vi "Serial Convert.vi"(8 "Range (V)":sgl=20.0 format="%#_13g", 11 "Raw serial buffer":string="\u0000\u0000\u0000\u0000\u0000\u0000\u0000\u0000\u0000\u0000\u0000\u0000\u0000\u0000\u0000\u0000\u0000\u0000") -> (0 "V6 (V)":sgl, 1 "V5 (V)":sgl, 2 "V4 (V)":sgl, 3 "V3 (V)":sgl, 4 "V7 (V)":sgl, 5 "V2 (V)":sgl, 6 "V8 (V)":sgl, 7 "V1 (V)":sgl)   [LabVIEW 2014]
panel:
  # "PN 20/11/2014"
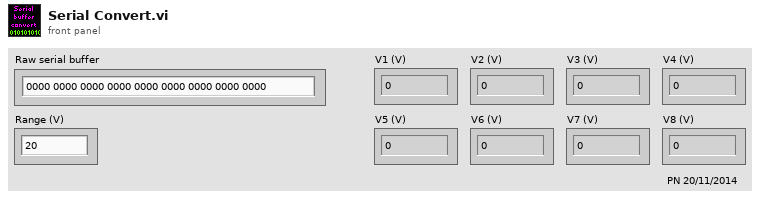
[diagram p1: front panel]
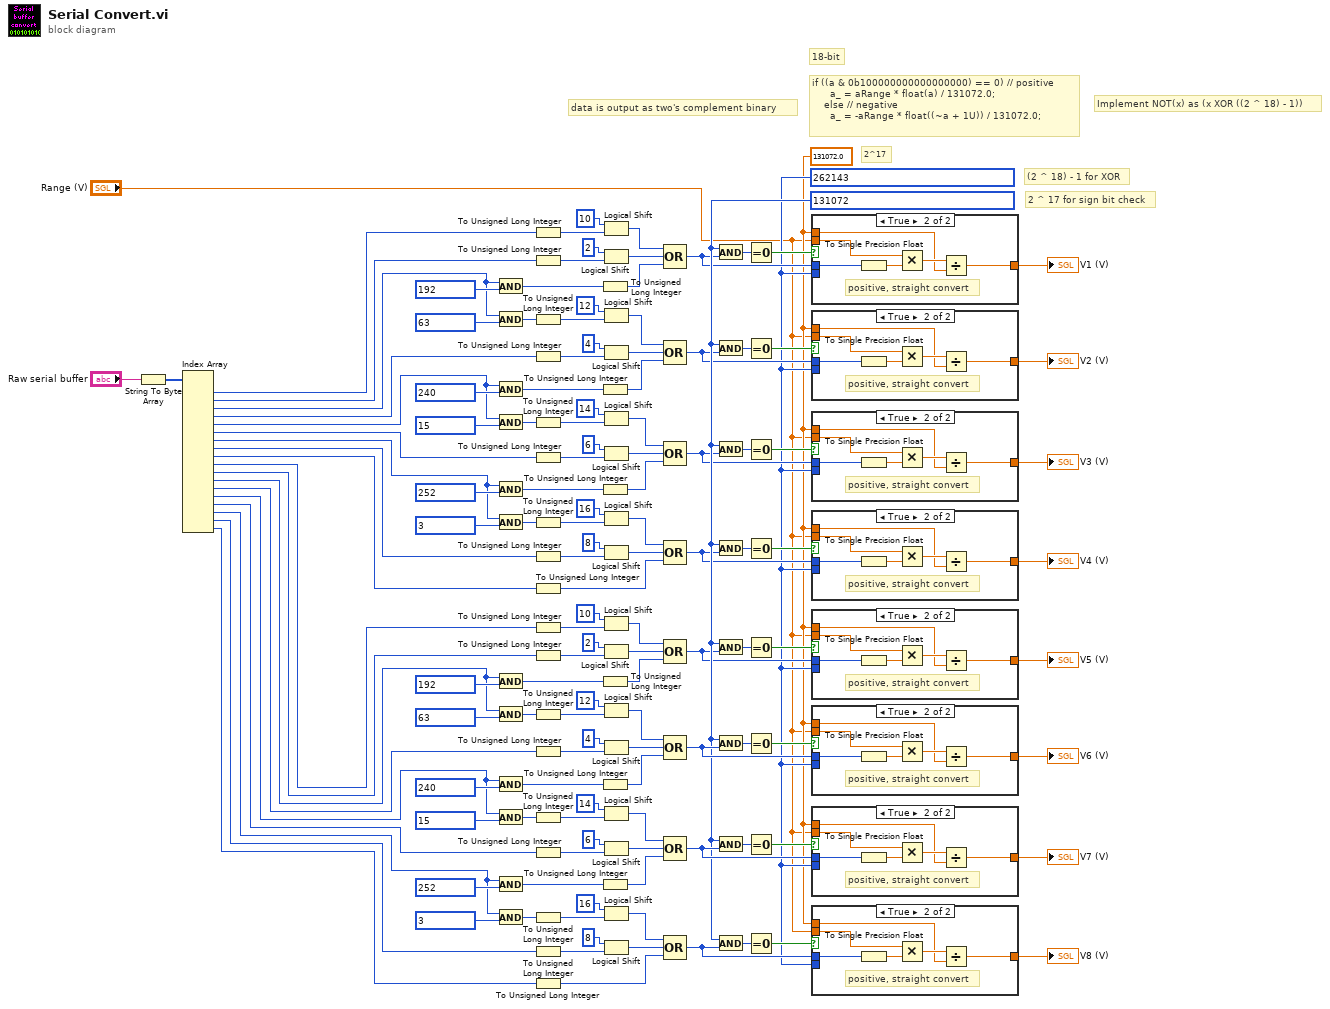
[diagram p0: block diagram]
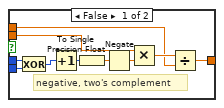
[diagram p2: hidden frame]
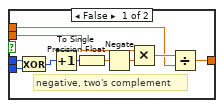
[diagram p3: hidden frame]
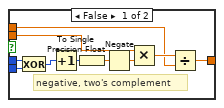
[diagram p4: hidden frame]
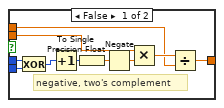
[diagram p5: hidden frame]
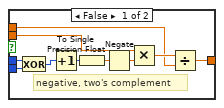
[diagram p6: hidden frame]
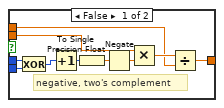
[diagram p7: hidden frame]
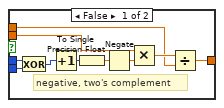
[diagram p8: hidden frame]
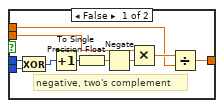
[diagram p9: hidden frame]
diagram:
  w3 = u32 262143
  w2 = sgl 131072.0
  w31 = u32 131072
  # "2 ^ 17 for sign bit check"
  # "(2 ^ 18) - 1 for XOR"
  # "Implement NOT(x) as (x XOR ((2 ^ 18) - 1))"
  # "18-bit"
  # "2^17"
  # "data is output as two's complement binary"
  # "if ((a & 0b100000000000000000) == 0) // positive\n      a_ = aRange * float(a) / 131072.0; \n    else // negative\n      a_ = -aRange * float((~a + 1U)) / 131072.0;"
  n1 = String To Byte Array(string="Raw serial buffer") -> (unsigned byte array=w131:u8[])
  n2 = Index Array(array=w131) -> (element #1=w135:u8, element #2=w132:u8, element #3=w122:u8, element #4=w118:u8, element #5=w109:u8, element #6=w104:u8, element #7=w96:u8, element #8=w91:u8, element #9=w87:u8, element #10=w30:u8, element #11=w29:u8, element #12=w28:u8, element #13=w27:u8, element #14=w26:u8, element #15=w25:u8, element #16=w24:u8, element #17=w23:u8, element #18=w22:u8)  [unwired: 18 in]
  n3 = And(x=w122, y=u8 192) -> (x .and. y?=w127:u8)
  n4 = And(x=w122, y=u8 63) -> (x .and. y?=w121:u8)
  n5 = And(x=w109, y=u8 240) -> (x .and. y?=w114:u8)
  n6 = And(x=w109, y=u8 15) -> (x .and. y?=w108:u8)
  n7 = And(x=w96, y=u8 252) -> (x .and. y?=w99:u8)
  n8 = And(x=w96, y=u8 3) -> (x .and. y?=w95:u8)
  n9 = And(x=w28, y=u8 192) -> (x .and. y?=w37:u8)
  n10 = And(x=w28, y=u8 63) -> (x .and. y?=w42:u8)
  n11 = And(x=w26, y=u8 240) -> (x .and. y?=w48:u8)
  n12 = And(x=w26, y=u8 15) -> (x .and. y?=w53:u8)
  n13 = And(x=w24, y=u8 252) -> (x .and. y?=w61:u8)
  n14 = And(x=w24, y=u8 3) -> (x .and. y?=w64:u8)
  n15 = To Unsigned Long Integer(number=w135) -> (unsigned 32bit integer=w130:u32)
  n16 = To Unsigned Long Integer(number=w132) -> (unsigned 32bit integer=w129:u32)
  n17 = To Unsigned Long Integer(number=w121) -> (unsigned 32bit integer=w120:u32)
  n18 = To Unsigned Long Integer(number=w118) -> (unsigned 32bit integer=w117:u32)
  n19 = To Unsigned Long Integer(number=w108) -> (unsigned 32bit integer=w106:u32)
  n20 = To Unsigned Long Integer(number=w104) -> (unsigned 32bit integer=w102:u32)
  n21 = To Unsigned Long Integer(number=w95) -> (unsigned 32bit integer=w93:u32)
  n22 = To Unsigned Long Integer(number=w91) -> (unsigned 32bit integer=w89:u32)
  n23 = To Unsigned Long Integer(number=w87) -> (unsigned 32bit integer=w86:u32)
  n24 = To Unsigned Long Integer(number=w30) -> (unsigned 32bit integer=w34:u32)
  n25 = To Unsigned Long Integer(number=w29) -> (unsigned 32bit integer=w35:u32)
  n26 = To Unsigned Long Integer(number=w42) -> (unsigned 32bit integer=w43:u32)
  n27 = To Unsigned Long Integer(number=w27) -> (unsigned 32bit integer=w45:u32)
  n28 = To Unsigned Long Integer(number=w53) -> (unsigned 32bit integer=w55:u32)
  n29 = To Unsigned Long Integer(number=w25) -> (unsigned 32bit integer=w58:u32)
  n30 = To Unsigned Long Integer(number=w64) -> (unsigned 32bit integer=w66:u32)
  n31 = To Unsigned Long Integer(number=w23) -> (unsigned 32bit integer=w69:u32)
  n32 = To Unsigned Long Integer(number=w22) -> (unsigned 32bit integer=w71:u32)
  n33 = To Unsigned Long Integer(number=w127) -> (unsigned 32bit integer=w126:u32)
  n34 = To Unsigned Long Integer(number=w114) -> (unsigned 32bit integer=w111:u32)
  n35 = To Unsigned Long Integer(number=w99) -> (unsigned 32bit integer=w98:u32)
  n36 = To Unsigned Long Integer(number=w37) -> (unsigned 32bit integer=w38:u32)
  n37 = To Unsigned Long Integer(number=w48) -> (unsigned 32bit integer=w51:u32)
  n38 = To Unsigned Long Integer(number=w61) -> (unsigned 32bit integer=w62:u32)
  n39 = Logical Shift(y=i16 10, x=w130) -> (x << y=w124:u32)
  n40 = Logical Shift(y=i16 2, x=w129) -> (x << y=w125:u32)
  n41 = Logical Shift(y=i16 12, x=w120) -> (x << y=w113:u32)
  n42 = Logical Shift(y=i16 4, x=w117) -> (x << y=w112:u32)
  n43 = Logical Shift(y=i16 14, x=w106) -> (x << y=w105:u32)
  n44 = Logical Shift(y=i16 6, x=w102) -> (x << y=w101:u32)
  n45 = Logical Shift(y=i16 16, x=w93) -> (x << y=w92:u32)
  n46 = Logical Shift(y=i16 8, x=w89) -> (x << y=w88:u32)
  n47 = Logical Shift(y=i16 10, x=w34) -> (x << y=w40:u32)
  n48 = Logical Shift(y=i16 2, x=w35) -> (x << y=w39:u32)
  n49 = Logical Shift(y=i16 12, x=w43) -> (x << y=w49:u32)
  n50 = Logical Shift(y=i16 4, x=w45) -> (x << y=w50:u32)
  n51 = Logical Shift(y=i16 14, x=w55) -> (x << y=w56:u32)
  n52 = Logical Shift(y=i16 6, x=w58) -> (x << y=w59:u32)
  n53 = Logical Shift(y=i16 16, x=w66) -> (x << y=w67:u32)
  n54 = Logical Shift(y=i16 8, x=w69) -> (x << y=w70:u32)
  n55 = Compound Arithmetic op=OR(w124, w125, w126) -> (w16:u32)
  n56 = Compound Arithmetic op=OR(w113, w112, w111) -> (w5:u32)
  n57 = Compound Arithmetic op=OR(w105, w101, w98) -> (w8:u32)
  n58 = Compound Arithmetic op=OR(w92, w88, w86) -> (w7:u32)
  n59 = Compound Arithmetic op=OR(w40, w39, w38) -> (w4:u32)
  n60 = Compound Arithmetic op=OR(w49, w50, w51) -> (w80:u32)
  n61 = Compound Arithmetic op=OR(w56, w59, w62) -> (w81:u32)
  n62 = Compound Arithmetic op=OR(w67, w70, w71) -> (w21:u32)
  n63 = And(x=w31, y=w16) -> (x .and. y?=w85:u32)
  n64 = And(x=w31, y=w5) -> (x .and. y?=w84:u32)
  n65 = And(x=w31, y=w8) -> (x .and. y?=w83:u32)
  n66 = And(x=w31, y=w7) -> (x .and. y?=w82:u32)
  n67 = And(x=w31, y=w4) -> (x .and. y?=w72:u32)
  n68 = And(x=w31, y=w80) -> (x .and. y?=w73:u32)
  n69 = And(x=w31, y=w81) -> (x .and. y?=w74:u32)
  n70 = And(x=w31, y=w21) -> (x .and. y?=w79:u32)
  n71 = Equal To 0?(x=w85) -> (x = 0?=w17:bool)
  n72 = Equal To 0?(x=w84) -> (x = 0?=w6:bool)
  n73 = Equal To 0?(x=w83) -> (x = 0?=w15:bool)
  n74 = Equal To 0?(x=w82) -> (x = 0?=w10:bool)
  n75 = Equal To 0?(x=w72) -> (x = 0?=w9:bool)
  n76 = Equal To 0?(x=w73) -> (x = 0?=w75:bool)
  n77 = Equal To 0?(x=w74) -> (x = 0?=w76:bool)
  n78 = Equal To 0?(x=w79) -> (x = 0?=w20:bool)
  n79 = case shown="True" w17 {
    tunnel: "Range (V)" -> [w143 w150]
    tunnel: w2 -> [w142 w148]
    tunnel: w16 -> [w138 w152]
    tunnel: [w141 w147] -> w18
    tunnel: w3 -> [w137 _]
    frame False {
      # "negative, two's complement"
      n80 = Exclusive Or(1:w137, 2:w138) -> (0:w139:u32)
      n81 = Increment(x=w139) -> (x+1=w144:u32)
      n82 = To Single Precision Float(number=w144) -> (single precision float=w146:sgl)
      n83 = Negate(x=w146) -> (-x=w140:sgl)
      n84 = Multiply(x=w143, y=w140) -> (x*y=w145:sgl)
      n85 = Divide(x=w145, y=w142) -> (x/y=w141:sgl)
    }
    frame True {
      # "positive, straight convert"
      n86 = To Single Precision Float(number=w152) -> (single precision float=w151:sgl)
      n87 = Multiply(x=w150, y=w151) -> (x*y=w149:sgl)
      n88 = Divide(x=w149, y=w148) -> (x/y=w147:sgl)
    }
  }
  "V1 (V)" <- w18
  n89 = case shown="True" w6 {
    tunnel: "Range (V)" -> [w159 w166]
    tunnel: w2 -> [w158 w164]
    tunnel: w5 -> [w154 w168]
    tunnel: [w157 w163] -> w13
    tunnel: w3 -> [w153 _]
    frame False {
      # "negative, two's complement"
      n90 = Exclusive Or(1:w153, 2:w154) -> (0:w155:u32)
      n91 = Increment(x=w155) -> (x+1=w160:u32)
      n92 = To Single Precision Float(number=w160) -> (single precision float=w162:sgl)
      n93 = Negate(x=w162) -> (-x=w156:sgl)
      n94 = Multiply(x=w159, y=w156) -> (x*y=w161:sgl)
      n95 = Divide(x=w161, y=w158) -> (x/y=w157:sgl)
    }
    frame True {
      # "positive, straight convert"
      n96 = To Single Precision Float(number=w168) -> (single precision float=w167:sgl)
      n97 = Multiply(x=w166, y=w167) -> (x*y=w165:sgl)
      n98 = Divide(x=w165, y=w164) -> (x/y=w163:sgl)
    }
  }
  "V2 (V)" <- w13
  n99 = case shown="True" w15 {
    tunnel: "Range (V)" -> [w175 w182]
    tunnel: w2 -> [w174 w180]
    tunnel: w8 -> [w170 w184]
    tunnel: [w173 w179] -> w14
    tunnel: w3 -> [w169 _]
    frame False {
      # "negative, two's complement"
      n100 = Exclusive Or(1:w169, 2:w170) -> (0:w171:u32)
      n101 = Increment(x=w171) -> (x+1=w176:u32)
      n102 = To Single Precision Float(number=w176) -> (single precision float=w178:sgl)
      n103 = Negate(x=w178) -> (-x=w172:sgl)
      n104 = Multiply(x=w175, y=w172) -> (x*y=w177:sgl)
      n105 = Divide(x=w177, y=w174) -> (x/y=w173:sgl)
    }
    frame True {
      # "positive, straight convert"
      n106 = To Single Precision Float(number=w184) -> (single precision float=w183:sgl)
      n107 = Multiply(x=w182, y=w183) -> (x*y=w181:sgl)
      n108 = Divide(x=w181, y=w180) -> (x/y=w179:sgl)
    }
  }
  "V3 (V)" <- w14
  n109 = case shown="True" w10 {
    tunnel: "Range (V)" -> [w191 w198]
    tunnel: w2 -> [w190 w196]
    tunnel: w7 -> [w186 w200]
    tunnel: [w189 w195] -> w12
    tunnel: w3 -> [w185 _]
    frame False {
      # "negative, two's complement"
      n110 = Exclusive Or(1:w185, 2:w186) -> (0:w187:u32)
      n111 = Increment(x=w187) -> (x+1=w192:u32)
      n112 = To Single Precision Float(number=w192) -> (single precision float=w194:sgl)
      n113 = Negate(x=w194) -> (-x=w188:sgl)
      n114 = Multiply(x=w191, y=w188) -> (x*y=w193:sgl)
      n115 = Divide(x=w193, y=w190) -> (x/y=w189:sgl)
    }
    frame True {
      # "positive, straight convert"
      n116 = To Single Precision Float(number=w200) -> (single precision float=w199:sgl)
      n117 = Multiply(x=w198, y=w199) -> (x*y=w197:sgl)
      n118 = Divide(x=w197, y=w196) -> (x/y=w195:sgl)
    }
  }
  "V4 (V)" <- w12
  n119 = case shown="True" w9 {
    tunnel: "Range (V)" -> [w207 w214]
    tunnel: w2 -> [w206 w212]
    tunnel: w4 -> [w202 w216]
    tunnel: [w205 w211] -> w11
    tunnel: w3 -> [w201 _]
    frame False {
      # "negative, two's complement"
      n120 = Exclusive Or(1:w201, 2:w202) -> (0:w203:u32)
      n121 = Increment(x=w203) -> (x+1=w208:u32)
      n122 = To Single Precision Float(number=w208) -> (single precision float=w210:sgl)
      n123 = Negate(x=w210) -> (-x=w204:sgl)
      n124 = Multiply(x=w207, y=w204) -> (x*y=w209:sgl)
      n125 = Divide(x=w209, y=w206) -> (x/y=w205:sgl)
    }
    frame True {
      # "positive, straight convert"
      n126 = To Single Precision Float(number=w216) -> (single precision float=w215:sgl)
      n127 = Multiply(x=w214, y=w215) -> (x*y=w213:sgl)
      n128 = Divide(x=w213, y=w212) -> (x/y=w211:sgl)
    }
  }
  "V5 (V)" <- w11
  n129 = case shown="True" w75 {
    tunnel: "Range (V)" -> [w223 w230]
    tunnel: w2 -> [w222 w228]
    tunnel: w80 -> [w218 w232]
    tunnel: [w221 w227] -> w77
    tunnel: w3 -> [w217 _]
    frame False {
      # "negative, two's complement"
      n130 = Exclusive Or(1:w217, 2:w218) -> (0:w219:u32)
      n131 = Increment(x=w219) -> (x+1=w224:u32)
      n132 = To Single Precision Float(number=w224) -> (single precision float=w226:sgl)
      n133 = Negate(x=w226) -> (-x=w220:sgl)
      n134 = Multiply(x=w223, y=w220) -> (x*y=w225:sgl)
      n135 = Divide(x=w225, y=w222) -> (x/y=w221:sgl)
    }
    frame True {
      # "positive, straight convert"
      n136 = To Single Precision Float(number=w232) -> (single precision float=w231:sgl)
      n137 = Multiply(x=w230, y=w231) -> (x*y=w229:sgl)
      n138 = Divide(x=w229, y=w228) -> (x/y=w227:sgl)
    }
  }
  "V6 (V)" <- w77
  n139 = case shown="True" w76 {
    tunnel: "Range (V)" -> [w239 w246]
    tunnel: w2 -> [w238 w244]
    tunnel: w81 -> [w234 w248]
    tunnel: [w237 w243] -> w78
    tunnel: w3 -> [w233 _]
    frame False {
      # "negative, two's complement"
      n140 = Exclusive Or(1:w233, 2:w234) -> (0:w235:u32)
      n141 = Increment(x=w235) -> (x+1=w240:u32)
      n142 = To Single Precision Float(number=w240) -> (single precision float=w242:sgl)
      n143 = Negate(x=w242) -> (-x=w236:sgl)
      n144 = Multiply(x=w239, y=w236) -> (x*y=w241:sgl)
      n145 = Divide(x=w241, y=w238) -> (x/y=w237:sgl)
    }
    frame True {
      # "positive, straight convert"
      n146 = To Single Precision Float(number=w248) -> (single precision float=w247:sgl)
      n147 = Multiply(x=w246, y=w247) -> (x*y=w245:sgl)
      n148 = Divide(x=w245, y=w244) -> (x/y=w243:sgl)
    }
  }
  "V7 (V)" <- w78
  n149 = case shown="True" w20 {
    tunnel: "Range (V)" -> [w255 w262]
    tunnel: w2 -> [w254 w260]
    tunnel: w21 -> [w250 w264]
    tunnel: [w253 w259] -> w19
    tunnel: w3 -> [w249 _]
    frame False {
      # "negative, two's complement"
      n150 = Exclusive Or(1:w249, 2:w250) -> (0:w251:u32)
      n151 = Increment(x=w251) -> (x+1=w256:u32)
      n152 = To Single Precision Float(number=w256) -> (single precision float=w258:sgl)
      n153 = Negate(x=w258) -> (-x=w252:sgl)
      n154 = Multiply(x=w255, y=w252) -> (x*y=w257:sgl)
      n155 = Divide(x=w257, y=w254) -> (x/y=w253:sgl)
    }
    frame True {
      # "positive, straight convert"
      n156 = To Single Precision Float(number=w264) -> (single precision float=w263:sgl)
      n157 = Multiply(x=w262, y=w263) -> (x*y=w261:sgl)
      n158 = Divide(x=w261, y=w260) -> (x/y=w259:sgl)
    }
  }
  "V8 (V)" <- w19
